vi "ccc_WriteError.vi"(8 "error in (no error)":errorcluster, 11 "Connection Info":T1) -> (0 "error out":errorcluster, 3 "Connection Info":T1)   [LabVIEW 2010]
uses:
  <vilib>/NI/STM/compatibility/stm_TCP Connection Info.ctl
  <vilib>/NI/STM/compatibility/stm_MetaDataElement.ctl
  NI_CCC.lvlib
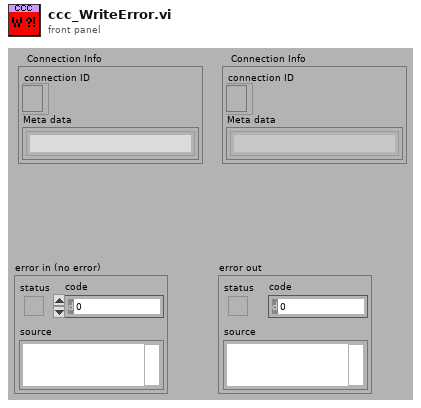
[diagram p1: front panel]
types:
  T1 = typedef "stm_TCP Connection Info.ctl" = cluster{"connection ID":refnum<k5>, "Meta data":T2[]}
  T2 = typedef "stm_MetaDataElement.ctl" = string
  T3 = typedef "NI STM.lvlib/TCP Connection Info.ctl" = cluster{"connection ID":refnum<k5>, "Meta data":T4[]}
  T4 = typedef "NI STM.lvlib/MetaDataElement.ctl" = string
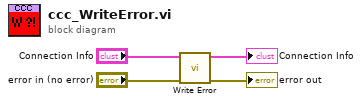
[diagram p0: block diagram]
diagram:
  n1 = call "Write Error.vi"("error in"="error in (no error)", "Connection Info In"="Connection Info") -> ("error out"=→"error out":errorcluster, "Connection Info Out"=→"Connection Info":T3)  [unwired: 8 in]
